vi "Initialize Console Options.vi"(8 "error in (no error)":errorcluster, 11 "Fancy Entry Console View in":refnum<class "Fancy Entry Console View.lvclass">) -> (0 "error out":errorcluster, 3 "Fancy Entry Console View out":refnum<class "Fancy Entry Console View.lvclass">)   [LabVIEW 2019, in "Fancy Entry Console View.lvclass"]
uses:
  <vilib>/gpm_packages/@cs/Car-wash/Source/Fancy Entry Console View/Fancy Entry Console View/Fancy Entry Console View.lvclass
  C:/Program Files/National Instruments/LabVIEW 2019/vi.lib/gpm_packages/@cs/Car-wash/Source/Entry Console View Definition/Entry Console View Definition/Entry Console View Definition.lvclass
  <vilib>/gpm_packages/@cs/Car-wash/Source/Entry Console View Definition/Entry Console View Definition/Entry Console View Definition.lvclass
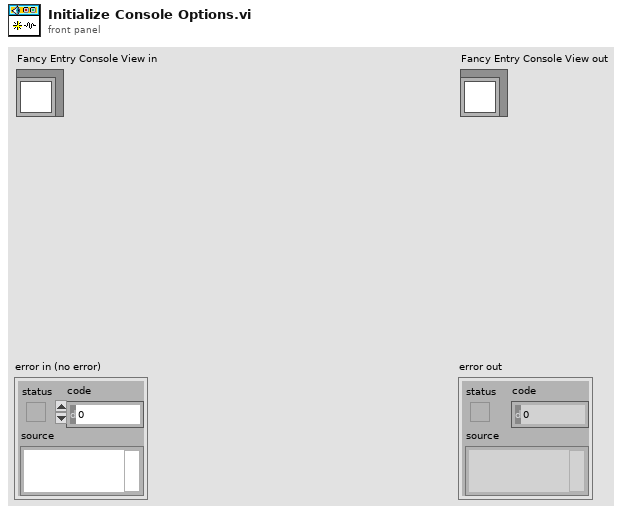
[diagram p1: front panel]
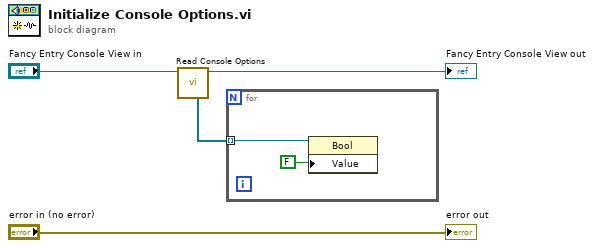
[diagram p0: block diagram]
diagram:
  n1 = call <vilib>:"Read Console Options.vi"("Entry Console View Definition in"="Fancy Entry Console View in") -> ("Entry Console View Definition out"=→"Fancy Entry Console View out":refnum<class "Fancy Entry Console View.lvclass">, "Console Options"=w1:refnum<vi>[])  [unwired: 9 in]
  n2 = for {
    tunnel: w1 -> [w6] mode=indexing
    n3 = property class="Bool"(reference=w6, "Value"=FALSE) -> ()  [unwired: 1 in, 2 out]
  }
  "error out" <- "error in (no error)"
